vi "Calc Shortest Difference.vi"(5 "Min Value":dbl=1023.0 format="%#_13g", 7 "Max Value":dbl=1023.0 format="%#_13g", 10 "Previous Real Position":dbl, 11 "New Real Position":dbl) -> (2 "Shortest Distance Out":dbl, 3 "Shortest Direction Out":dbl)   [LabVIEW 2023, in "TShirtWork-SwerveDrive_ACT_ts.lvlib"]
uses:
  TShirtWork-SwerveDrive_ACT_ts.lvlib
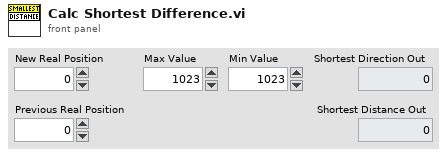
[diagram p1: front panel]
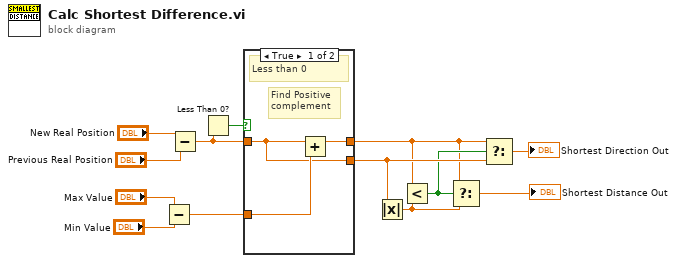
[diagram p0: block diagram]
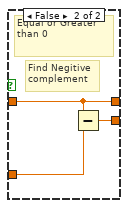
[diagram p2: hidden frame]
diagram:
  n1 = Subtract(x="Max Value", y="Min Value") -> (x-y=w1:dbl)
  n2 = Subtract(x="New Real Position", y="Previous Real Position") -> (x-y=w10:dbl)
  n3 = Less Than 0?(x=w10) -> (x < 0?=w11:bool)
  n4 = case shown="True" w11 {
    tunnel: w10 -> [w14 w19]
    tunnel: w1 -> [w16 w17]
    tunnel: [w15 w19] -> w4
    tunnel: [w14 w18] -> w8
    frame True {
      # "Find Positive\ncomplement"
      # "Less than 0"
      n5 = Add(x=w14, y=w16) -> (x+y=w15:dbl)
    }
    frame False {
      # "Find Negitive\ncomplement"
      # "Equal or Greater than 0"
      n6 = Subtract(x=w19, y=w17) -> (x-y=w18:dbl)
    }
  }
  n7 = Absolute Value(x=w8) -> (abs(x)=w7:dbl)
  n8 = Less?(x=w4, y=w7) -> (x < y?=w5:bool)
  n9 = Select(t=w4, s=w5, f=w7) -> (s? t:f=→"Shortest Distance Out":dbl)
  n10 = Select(t=w4, s=w5, f=w8) -> (s? t:f=→"Shortest Direction Out":dbl)
